vi "AddToPower.vi"(1 "MODE":i32(knob) scale=0.0..2.0) -> (0 "AddToPower":dbl)   [LabVIEW 2013]
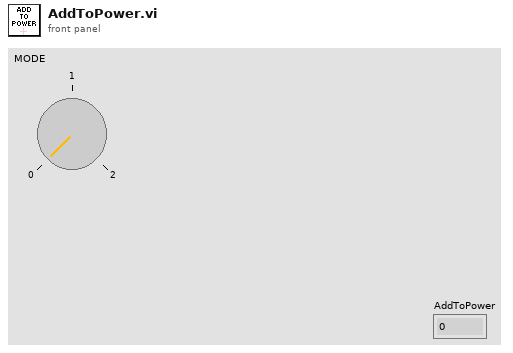
[diagram p1: front panel]
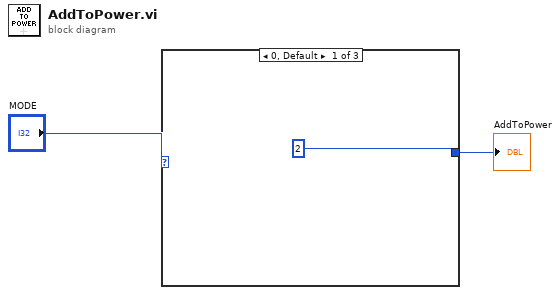
[diagram p0: block diagram]
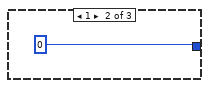
[diagram p2: hidden frame]
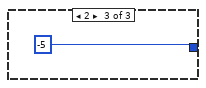
[diagram p3: hidden frame]
diagram:
  n1 = case shown="0, Default" "MODE" {
    tunnel: [2 0 -5] -> w1
    frame 0, Default {
    }
    frame 1 {
    }
    frame 2 {
    }
  }
  "AddToPower" <- w1
